vi "Snd Read Wave File+.vi"(8 "error in (no error)":errorcluster, 11 "wave file path":path) -> (0 "error out":errorcluster, 2 "sound format":T1, 3 "wave file path out":path, 4 "stereo 16-bit":i16[][](array[numeric]), 5 "mono 16-bit":i16[](array[numeric]), 6 "stereo 8-bit":u8[][](array[numeric]), 7 "mono 8-bit":u8[](array[numeric]))   [LabVIEW 2017]
doc: "This vi retrieves sound information from a PC waveform audio file (.wav). The information returned includes both waveform data and sound format data which is necessary for configuring a sound device to play the waveform."
uses:
  <vilib>/addons/Sound and Vibration/Order Analysis/Example Support/Demo VI/Start-Up Kit/File Access/Sound Format+.ctl
panel:
  in  "sound format":T1
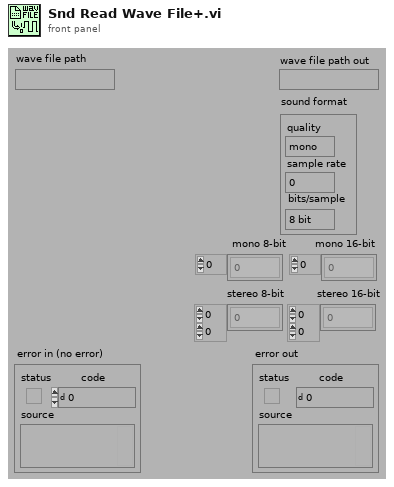
[diagram p1: front panel]
types:
  T1 = typedef "Sound Format+.ctl" = cluster{"quality":enum16{"mono", "stereo"}, "sample rate":u32, "bits/sample":enum16{"8 bit", "16 bit"}}
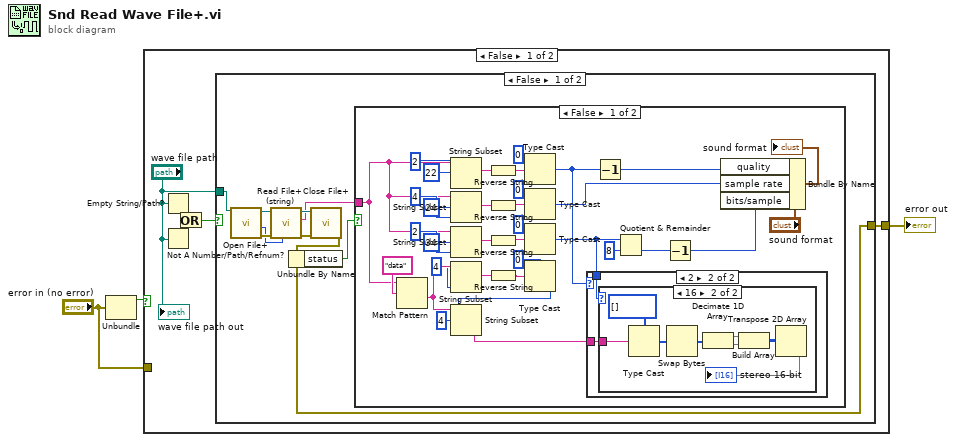
[diagram p0: block diagram]
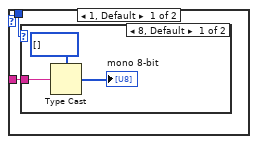
[diagram p2: hidden frame]
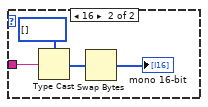
[diagram p3: hidden frame]
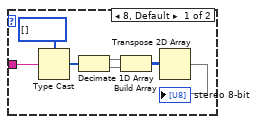
[diagram p4: hidden frame]
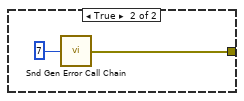
[diagram p6: hidden frame]
diagram:
  n1 = Unbundle("error in (no error)") -> ("status"=w2:bool)  [unwired: 2 out]
  n2 = case shown="False" w2 {
    tunnel: "error in (no error)" -> [_ w80]
    tunnel: [w4 w80] -> w1
    frame False {
      n3 = Empty String/Path?(string/path="wave file path") -> (empty?=w8:bool)
      n4 = Not A Number/Path/Refnum?(number/path/refnum="wave file path") -> (NaN/Path/Refnum?=w7:bool)
      n5 = Or(x=w8, y=w7) -> (x .or. y?=w6:bool)
      n6 = case shown="False" w6 {
        tunnel: "wave file path" -> [w12 _]
        tunnel: [w11 w78] -> w4
        frame False {
          n7 = call <vilib>:"Open File+.vi"("file path (\" \")"=w12) -> ("error out"=w15:errorcluster, "file size (bytes)"=w13:i32, "refnum"=w17:refnum<file>)  [unwired: 7 in, 1 out]
          n8 = call <vilib>:"Read File+ (string).vi"("count"=w13, "error in (no error)"=w15, "refnum"=w17) -> ("error out"=w14:errorcluster, "string"=w9:string, "dup refnum"=w16:refnum<file>)  [unwired: 4 in, 2 out]
          n9 = call <vilib>:"Close File+.vi"("error in (no error)"=w14, "refnum"=w16) -> ("error out"=w11:errorcluster)  [unwired: 3 in, 2 out]
          n10 = Unbundle By Name(w11) -> ("status"=w10:bool)
          n11 = case shown="False" w10 {
            tunnel: w9 -> [w25 _]
            frame False {
              n12 = Match Pattern(string=w25, regular expression="data") -> (after substring=w51:string)  [unwired: 1 in, 3 out]
              n13 = String Subset(string=w25, offset (0)=22, length (rest)=2 ("length")) -> (substring=w40:string)
              n14 = String Subset(string=w25, offset (0)=24, length (rest)=4 ("length")) -> (substring=w38:string)
              n15 = String Subset(string=w25, offset (0)=34, length (rest)=2 ("length")) -> (substring=w36:string)
              n16 = String Subset(string=w51, length (rest)=4 ("length")) -> (substring=w34:string)  [unwired: 1 in]
              n17 = Reverse String(1:w40) -> (0:w39:string)
              n18 = Reverse String(1:w38) -> (0:w37:string)
              n19 = Reverse String(1:w36) -> (0:w35:string)
              n20 = Reverse String(1:w34) -> (0:w31:string)
              n21 = Type Cast(type=u16 0, x=w39) -> (*(type *) &x=w23:u16)
              n22 = Type Cast(type=u32 0, x=w37) -> (*(type *) &x=w24:u32)
              n23 = Type Cast(type=u16 0, x=w35) -> (*(type *) &x=w20:u16)
              n24 = Type Cast(type=u32 0, x=w31) -> (*(type *) &x=w30:u32)
              n25 = String Subset(string=w51, offset (0)=4, length (rest)=w30) -> (substring=w29:string)
              n26 = case shown="2" w23 {
                tunnel: w20 -> [w53 w62]
                tunnel: w29 -> [w52 w61]
                frame 1, Default {
                  n27 = case shown="8, Default" w53 {
                    tunnel: w52 -> [w56 w60]
                    frame 8, Default {
                      n28 = Type Cast(type=u8[] [], x=w56) -> (*(type *) &x=→"mono 8-bit":u8[])
                    }
                    frame 16 {
                      n29 = Type Cast(type=i16[] [], x=w60) -> (*(type *) &x=w58:i16[])
                      n30 = Swap Bytes(anything=w58) -> (byte swapped=→"mono 16-bit":i16[])
                    }
                  }
                }
                frame 2 {
                  n31 = case shown="16" w62 {
                    tunnel: w61 -> [w69 w77]
                    frame 8, Default {
                      n32 = Type Cast(type=u8[] [], x=w69) -> (*(type *) &x=w64:u8[])
                      n33 = Decimate 1D Array(w64) -> (w65:u8[], w66:u8[])
                      n34 = Build Array(w65, w66) -> (w67:u8[][])
                      n35 = Transpose 2D Array(2D array=w67) -> (transposed array=→"stereo 8-bit":u8[][])
                    }
                    frame 16 {
                      n36 = Type Cast(type=i16[] [], x=w77) -> (*(type *) &x=w75:i16[])
                      n37 = Swap Bytes(anything=w75) -> (byte swapped=w74:i16[])
                      n38 = Decimate 1D Array(w74) -> (w73:i16[], w72:i16[])
                      n39 = Build Array(w73, w72) -> (w71:i16[][])
                      n40 = Transpose 2D Array(2D array=w71) -> (transposed array=→"stereo 16-bit":i16[][])
                    }
                  }
                }
              }
              n41 = Decrement(x=w23) -> (x-1=w22:u16)
              n42 = Quotient & Remainder(x=w20, y=u16 8) -> (floor(x/y)=w18:u16)  [unwired: 1 out]
              n43 = Decrement(x=w18) -> (x-1=w21:u16)
              n44 = Bundle By Name(cluster="sound format", "quality"=w22, "sample rate"=w24, "bits/sample"=w21) -> (→"sound format":T1)
            }
            frame True {
            }
          }
        }
        frame True {
          n45 = call <vilib>:"Snd Gen Error Call Chain.vi"("error code"=7) -> ("error out"=w78:errorcluster)
        }
      }
      "wave file path out" <- "wave file path"
    }
    frame True {
    }
  }
  "error out" <- w1
